vi "Create SimpleText Paragraph.vi"(8 "error in (no error)":errorcluster, 10 "simpleText":string, 11 "ooCalc in":refnum<class "ooCalc.lvclass">) -> (0 "error out":errorcluster, 2 "SimpleTextParagraph":refnum<k24>, 3 "ooCalc out":refnum<class "ooCalc.lvclass">)   [LabVIEW 2009, in "ooCalc.lvclass"]
uses:
  ooCalc.lvclass
  C:/Projets/LAVAG/OpenOfficeRGT/AODL/DLLs/AODL.dll
  ooCalc.lvclass/ooCalc.ctl
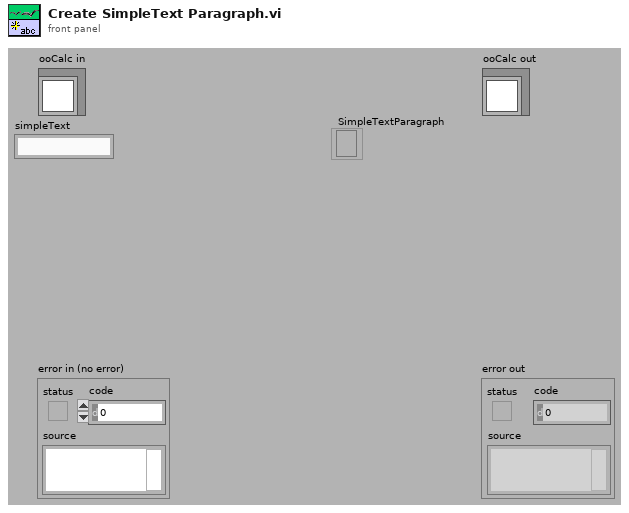
[diagram p1: front panel]
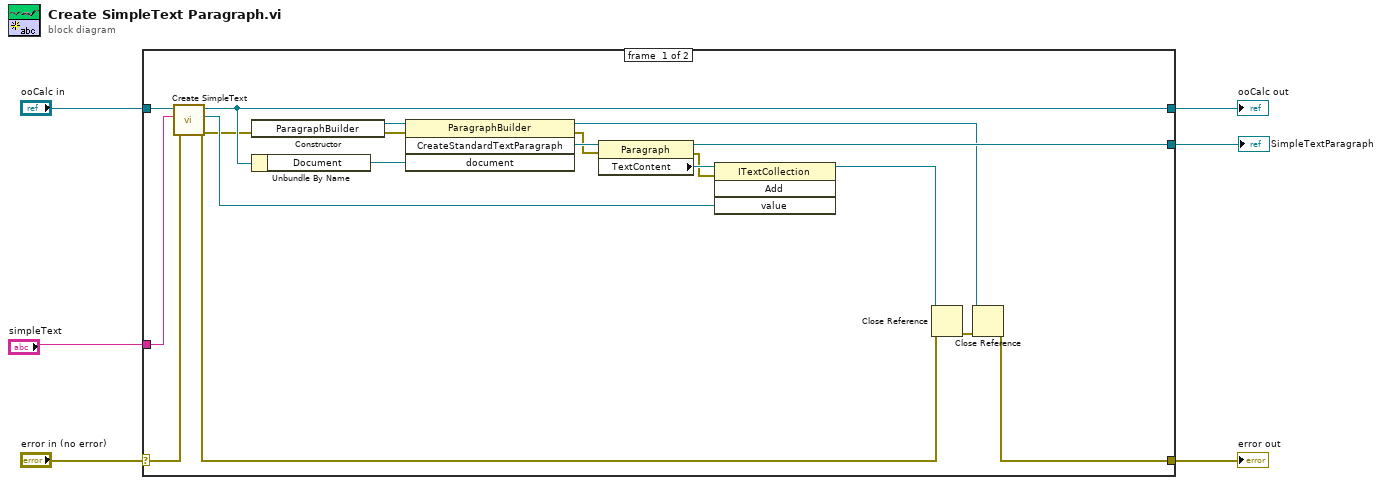
[diagram p0: block diagram]
diagram:
  n1 = case shown="No Error" "error in (no error)" {
    selector: "error in (no error)" -> [w17 w26]
    tunnel: [w7 w26] -> w5
    tunnel: [w18 w25] -> w3
    tunnel: "ooCalc in" -> [w19 w25]
    tunnel: "simpleText" -> [w15 _]
    tunnel: [w20 _] -> w1
    frame #0 {
      n2 = call-dynamic "Create SimpleText.vi"("error in (no error)"=w17, "simpleText"=w15, "ooDocument"=w19) -> ("error out"=w10:errorcluster, "SimpleText"=w16:refnum<k24>, "ooDocument out"=w18:refnum<class "ooCalc.lvclass">)  [unwired: 6 in]
      n3 = constructor class="ParagraphBuilder"(error in=w10) -> (reference out=w23:refnum<k24>, error out=w24:errorcluster)  [unwired: 2 in, 1 out]
      n4 = Unbundle By Name(w18) -> ("Document"=w21:refnum<k24>)
      n5 = invoke class="ParagraphBuilder" method="CreateStandardTextParagraph"(reference=w23, error in=w24, "document"=w21) -> (reference out=w8:refnum<k24>, error out=w12:errorcluster, "CreateStandardTextParagraph"=w13:refnum<k24>)  [unwired: 1 in, 1 out]
      n6 = property class="Paragraph"(reference=w13, error in=w12) -> (reference out=w20:refnum<k24>, error out=w11:errorcluster, "TextContent"=w22:refnum<k24>)
      n7 = invoke class="ITextCollection" method="Add"(reference=w22, error in=w11, "value"=w16) -> (reference out=w9:refnum<k24>)  [unwired: 1 in, 3 out]
      n8 = Close Reference(reference=w9, error in (no error)=w10) -> (error out=w14:errorcluster)
      n9 = Close Reference(reference=w8, error in (no error)=w14) -> (error out=w7:errorcluster)
    }
    frame #1 {
    }
  }
  "error out" <- w5
  "ooCalc out" <- w3
  "SimpleTextParagraph" <- w1
